vi "Read From CSV.vi"(8 "Error In":errorcluster, 11 "Spreadsheet path (.csv)":path=path "C:/Users/husmith/Desktop/MyData.csv") -> (0 "Error Out":errorcluster, 3 "Data":dbl[][](array[numeric]))   [LabVIEW 2017]
uses:
  <vilib>/Utility/file.llb/Read Delimited Spreadsheet (string).vi
  <vilib>/Utility/file.llb/Read Delimited Spreadsheet (DBL).vi
panel:
  in  "Headers?":bool
  out "String Display":string[][](array[string])
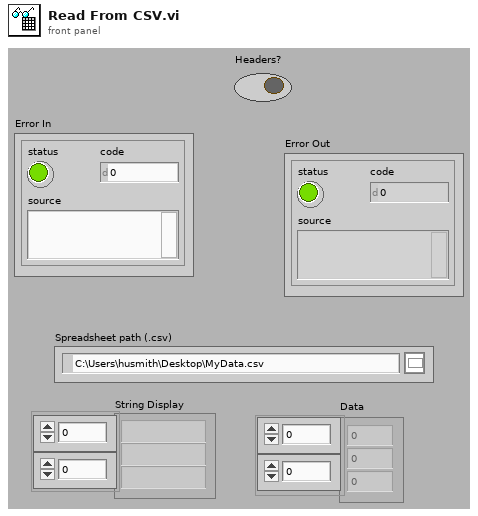
[diagram p1: front panel]
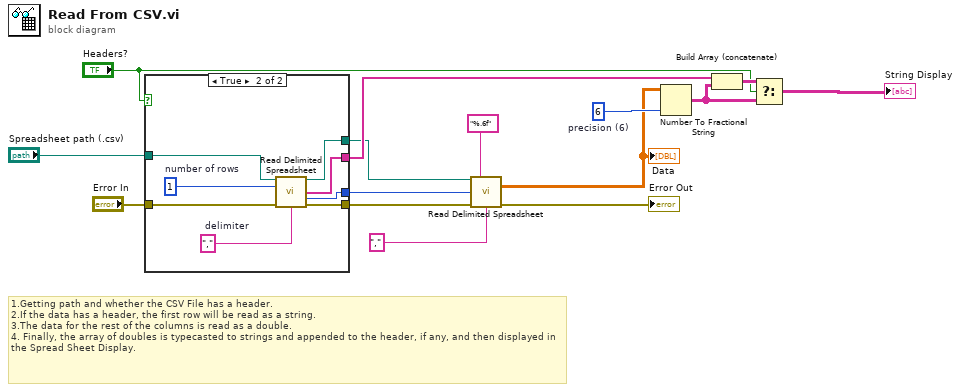
[diagram p0: block diagram]
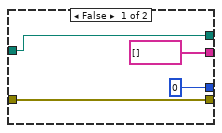
[diagram p2: hidden frame]
diagram:
  w10 = i16 6  # precision (6)
  # "1.Getting path and whether the CSV File has a header.\n2.If the data has a header, the first row will be read as a string.\n3.The data for the rest of the columns is read as a double.\n4. Finally, the array of doubles is typecasted to strings and appended to the header, if any, and then displayed in the Spread Sheet Display."
  n1 = case shown="True" "Headers?" {
    tunnel: "Spreadsheet path (.csv)" -> [w17 w27]
    tunnel: [string[] [] ("first row") w23] -> w14
    tunnel: [0 ("mark after read (chars.)") w22] -> w6
    tunnel: [w17 w26] -> w9
    tunnel: [w16 w21] -> w1
    tunnel: "Error In" -> [w16 w20]
    frame False {
    }
    frame True {
      w25 = 1  # number of rows
      w24 = ","  # delimiter
      n2 = call-poly <vilib>:"Read Delimited Spreadsheet.vi"("file path (dialog if empty)"=w27, "number of rows (all:-1)"=w25, "error in (no error)"=w20, "delimiter (\\t)"=w24) -> ("new file path (Not A Path if cancelled)"=w26:path, "first row"=w23:string[], "mark after read (chars.)"=w22:i32, "error out"=w21:errorcluster)  [unwired: 6 in, 2 out]
    }
  }
  n3 = call-poly <vilib>:"Read Delimited Spreadsheet.vi"("file path (dialog if empty)"=w9, "format (%.3f)"="%.6f", "start of read offset (chars.:0)"=w6, "error in (no error)"=w1, "delimiter (\\t)"="," ("delimiter (\\t)")) -> ("all rows"=w8:dbl[][], "error out"=→"Error Out":errorcluster)  [unwired: 5 in, 4 out]
  "Data" <- w8
  n4 = Number To Fractional String(number=w8, precision (6)=w10) -> (F-format string=w11:string[][])  [unwired: 2 in]
  n5 = Build Array (concatenate)(w14, w11) -> (w13:string[][])
  n6 = Select(t=w13, s="Headers?", f=w11) -> (s? t:f=→"String Display":string[][])
